vi "Wake up Load detect HL.vi"(8 "error in":errorcluster, 9 "Overload time":dbl, 10 "Overload threshold":dbl, 11 "Detecting speed":dbl) -> (0 "error out":errorcluster)   [LabVIEW 2020, in "Motherboard loading.lvlib"]
doc: "Continue require loadpercentage from motherboard\n_____\nCreated using DQMH Event Scripter 6.1.0.128."
uses:
  Motherboard loading.lvlib
  Wake up Load detect HL Argument--cluster.ctl
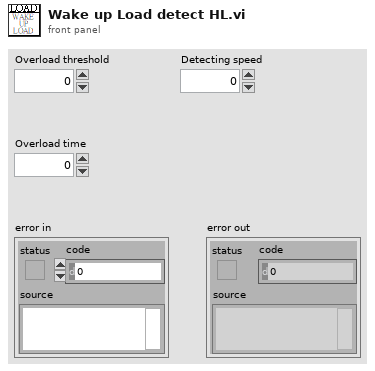
[diagram p1: front panel]
types:
  T1 = typedef "Motherboard loading.lvlib/Wake up Load detect HL Argument--cluster.ctl" = cluster{"Overload threshold":dbl, "Overload time":dbl, "Detecting speed":dbl}
  T2 = typedef "Motherboard loading.lvlib/Request Events--cluster.ctl" = cluster{"Stop Module":refnum<user-event>, "Show Panel":refnum<user-event>, "Hide Panel":refnum<user-event>, "Get Module Execution Status":refnum<user-event>, "Show Diagram":refnum<user-event>, "Start acquisition":refnum<user-event>, "Wake up Load detect HL":refnum<user-event>, "Put Load update HL to sleep":refnum<user-event>, "Stop acquisition":refnum<user-event>}
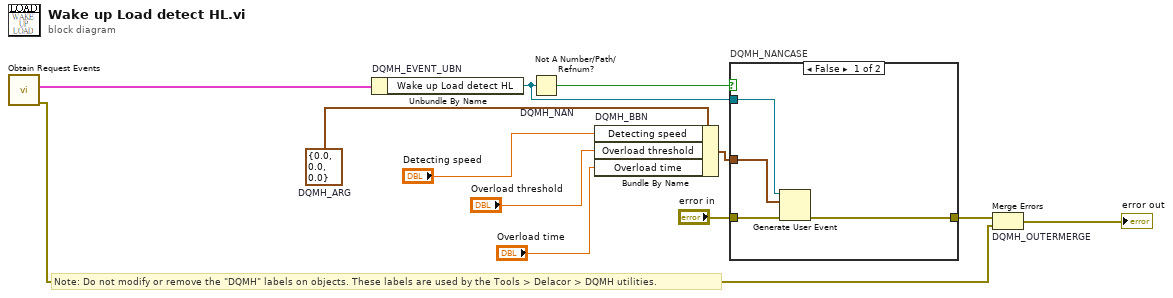
[diagram p0: block diagram]
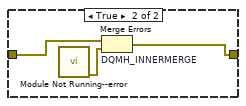
[diagram p2: hidden frame]
diagram:
  w6 = T1 {"Overload threshold"=0.0, "Overload time"=0.0, "Detecting speed"=0.0}  # DQMH_ARG
  # "Note: Do not modify or remove the \"DQMH\" labels on objects. These labels are used by the Tools > Delacor > DQMH utilities."
  n1 = call "Obtain Request Events.vi"() -> ("error out"=w3:errorcluster, "Motherboard loading Request Events"=w2:T2)  [unwired: 10 in]
  n2 = Unbundle By Name "DQMH_EVENT_UBN"(w2) -> ("Wake up Load detect HL"=w8:refnum<user-event>)
  n3 = Not A Number/Path/Refnum? "DQMH_NAN"(number/path/refnum=w8) -> (NaN/Path/Refnum?=w9:bool)
  n4 = Bundle By Name "DQMH_BBN"(cluster=w6, "Detecting speed"="Detecting speed", "Overload threshold"="Overload threshold", "Overload time"="Overload time") -> (w10:T1)
  n5 = case "DQMH_NANCASE" shown="False" w9 {
    tunnel: "error in" -> [w16 w19]
    tunnel: [w15 w18] -> w7
    tunnel: w8 -> [w14 _]
    tunnel: w10 -> [w13 _]
    frame False {
      n6 = Generate User Event(user event=w14, event data cluster=w13, error in=w16) -> (error out=w15:errorcluster)  [unwired: 1 in, 1 out]
    }
    frame True {
      n7 = call "Module Not Running--error.vi"() -> ("error out"=w17:errorcluster)  [unwired: 11 in]
      n8 = Merge Errors "DQMH_INNERMERGE"(w19, w17) -> (w18:errorcluster)
    }
  }
  n9 = Merge Errors "DQMH_OUTERMERGE"(w7, w3) -> (→"error out":errorcluster)
